vi "Threshold.vi"(6 "Default value":dbl, 9 "Threshold value":dbl, 11 "Input data values":dbl[](array[numeric])) -> (3 "Thresholded data values":dbl[](array[numeric]))   [LabVIEW 2012]
doc: "Compares data to threshold value, if data is less than the threshold value, the output data is the default value."
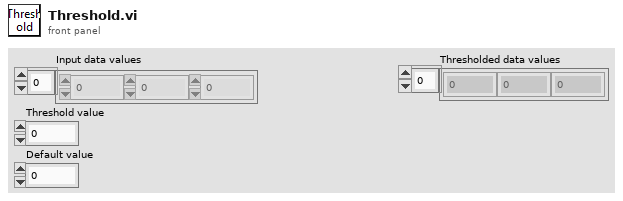
[diagram p1: front panel]
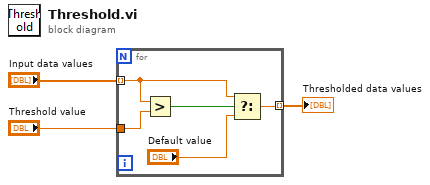
[diagram p0: block diagram]
diagram:
  n1 = for {
    tunnel: "Threshold value" -> [w8]
    tunnel: "Input data values" -> [w6] mode=indexing
    tunnel: [w4] -> w1 mode=indexing
    n2 = Greater?(x=w6, y=w8) -> (0:w7:bool)
    n3 = Select(t=w6, s=w7, f="Default value") -> (s? t:f=w4:dbl)
  }
  "Thresholded data values" <- w1
